vi "Add Item to Tree.vi"(0 "Parent Tag Name In":string, 1 "TreeControl in":refnum<vi>, 5 "File/Folder Names Array":string[](array[string]), 9 "variant in":variant, 11 "error in (no error)":errorcluster) -> (4 "Current File/Folder Name Out":string, 6 "Dup File/Folder Names Array":string[](array[string]), 10 "variant out":variant, 15 "error out":errorcluster)   [LabVIEW 2017]
panel:
  out "Navigate Tree:Get Path":string[](array[string])
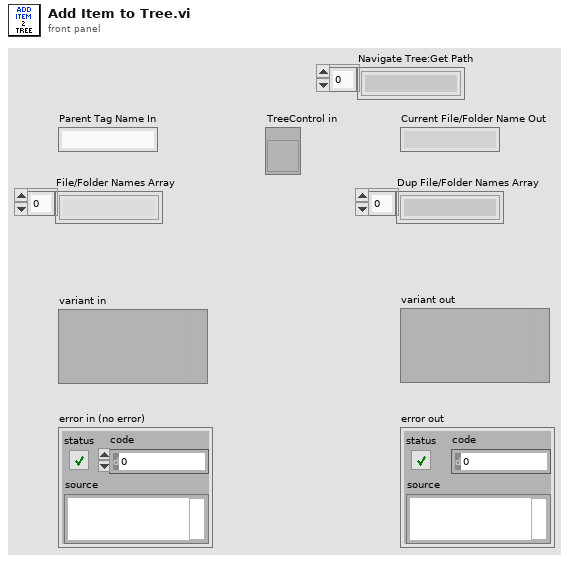
[diagram p1: front panel]
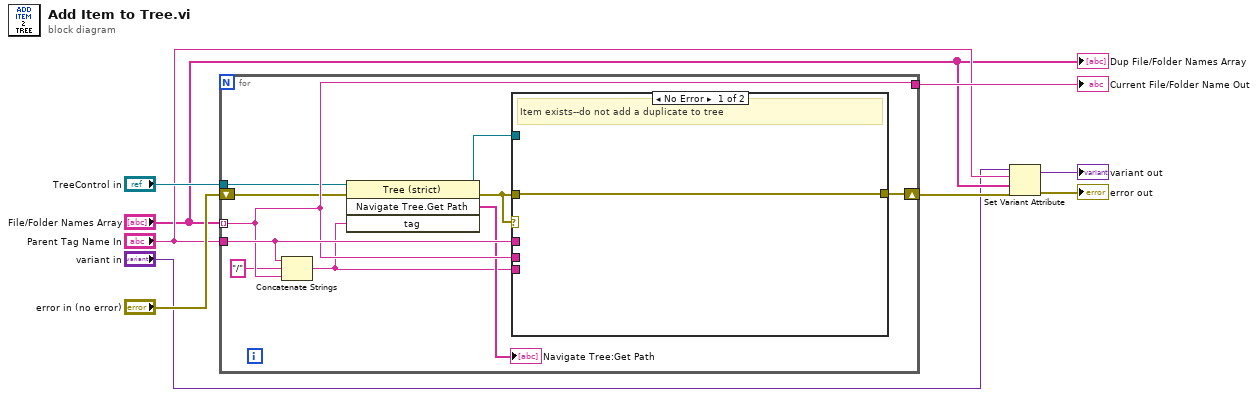
[diagram p0: block diagram]
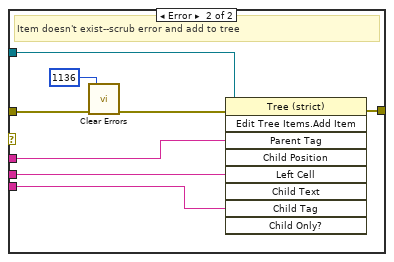
[diagram p2: hidden frame]
diagram:
  n1 = for {
    tunnel: "File/Folder Names Array" -> [w17] mode=indexing
    tunnel: "Parent Tag Name In" -> [w18]
    shift-right: [w19] -> w5
    shift-left: "error in (no error)" -> [w12]
    tunnel: [w17] -> w9
    tunnel: "TreeControl in" -> [w13]
    # "Add Folders"
    n2 = Concatenate Strings(w18, "/" ("string"), w17) -> (w14:string)
    n3 = invoke on="Invoke Node" class="Tree (strict)" method="Navigate Tree.Get Path"(reference=w13, error in=w12, "tag"=w14) -> (reference out=w11:refnum<vi>, error out=w10:errorcluster, "Navigate Tree:Get Path"=→"Navigate Tree:Get Path":string[])  [unwired: 1 in, 1 out]
    n4 = case shown="No Error" w10 {
      tunnel: [w20 w28] -> w19
      tunnel: w18 -> [_ w27]
      tunnel: w17 -> [_ w26]
      tunnel: w14 -> [_ w25]
      tunnel: w10 -> [w20 w23]
      tunnel: w11 -> [_ w21]
      frame No Error {
        # "Item exists--do not add a duplicate to tree"
      }
      frame Error {
        # "Item doesn't exist--scrub error and add to tree"
        n5 = call <vilib>:"Clear Errors.vi"("error in (no error)"=w23, "specific error code to clear (0: all)"=1136) -> ("error out"=w22:errorcluster)  [unwired: 4 in, 1 out]
        n6 = invoke on="Invoke Node" class="Tree (strict)" method="Edit Tree Items.Add Item"(reference=w21, error in=w22, "Parent Tag"=w27, "Left Cell"=w26, "Child Tag"=w25) -> (error out=w28:errorcluster)  [unwired: 4 in, 8 out]
      }
    }
  }
  "Current File/Folder Name Out" <- w9
  n7 = Set Variant Attribute(Variant="variant in", name="Parent Tag Name In", value="File/Folder Names Array", error in=w5) -> (Variant out=→"variant out":variant, error out=→"error out":errorcluster)  [unwired: 1 out]
  "Dup File/Folder Names Array" <- "File/Folder Names Array"
